vi "create.vi"(6 "Assets":string[](array[string]), 8 "error in (no error)":errorcluster, 9 "Start Time":timestamp format="%<%x %.3X>T", 10 "Title":string, 11 "Nominal Client":refnum<class "Nominal Client.lvclass">) -> (0 "error out":errorcluster, 3 "Run out":refnum<class "Run.lvclass">)   [LabVIEW 2020, in "Run.lvclass"]
uses:
  Run.lvclass
  Nominal Client/Nominal Client.lvclass
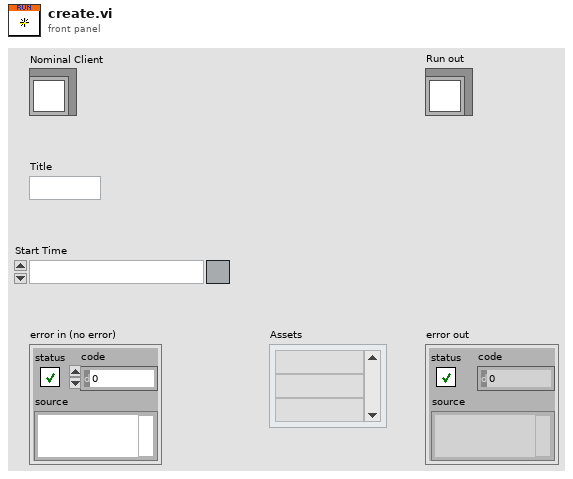
[diagram p1: front panel]
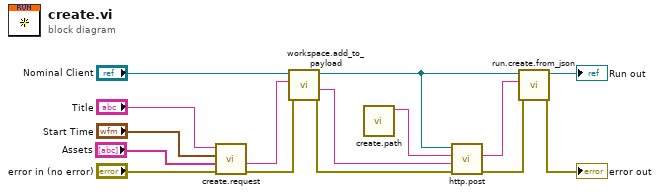
[diagram p0: block diagram]
diagram:
  n1 = call "create.request.vi"("error in"="error in (no error)", "Assets"="Assets", "Start Time"="Start Time", "Title"="Title") -> ("error out"=w3:errorcluster, "Request"=w4:string)  [unwired: 6 in]
  n2 = call "workspace.add_to_payload.vi"("error in"=w3, "JSON payload in"=w4, "Nominal Client in"="Nominal Client") -> ("error out"=w2:errorcluster, "JSON payload out"=w1:string, "Nominal Client out"=w5:refnum<class "Nominal Client.lvclass">)  [unwired: 6 in]
  n3 = call "create.path.vi"() -> ("Path"=w12:string)  [unwired: 11 in]
  n4 = call "http.post.vi"("error in"=w2, "Request body"=w1, "Path"=w12, "Nominal Client in"=w5) -> ("error out"=w9:errorcluster, "Response"=w10:string)  [unwired: 5 in, 1 out]
  n5 = call "run.create.from_json.vi"("error in"=w9, "JSON"=w10, "Nominal Client"=w5) -> ("error out"=→"error out":errorcluster, "Run out"=→"Run out":refnum<class "Run.lvclass">)  [unwired: 7 in]
